vi "_Read CSM Log Filter Rules - v1.0.vi"(7 "Section Name":string="LogFilterRules", 8 "error in (no error)":errorcluster, 11 "LabVIEW-Config.lvlib:LabVIEW-Config.lvclass":refnum<class "LabVIEW-Config.lvclass">) -> (0 "error out":errorcluster, 1 "Rules-v1":T1, 2 "Key Names":string[](array[string]), 3 "Config out":refnum<class "LabVIEW-Config.lvclass">)   [LabVIEW 2017, in "INI-Static-Variable-Support.lvlib"]
uses:
  INI-Static-Variable-Support.lvlib
  LabVIEW-Config/LabVIEW-Config.lvclass
  <userlib>/_NEVSTOP/Communicable State Machine(CSM)/_Support/Typedef/_CSM_GlobalLog Filter Rules - v1.0.ctl
  <userlib>/_NEVSTOP/Communicable State Machine(CSM)/_Support/Typedef/_CSM_GlobalLog_MSG_TYPE.ctl
  <userlib>/_NEVSTOP/Communicable State Machine(CSM)/_Support/Typedef/_CSM_GlobalLog_STATE_TYPE.ctl
  LabVIEW-Config/Read Array Key (String).vi
  <userlib>/_NEVSTOP/Communicable State Machine(CSM)/Communicable State Machine.lvlib
  <userlib>/_NEVSTOP/Communicable State Machine(CSM)/addons/API-String-Arugments-Support/API String Arguments Support.lvlib
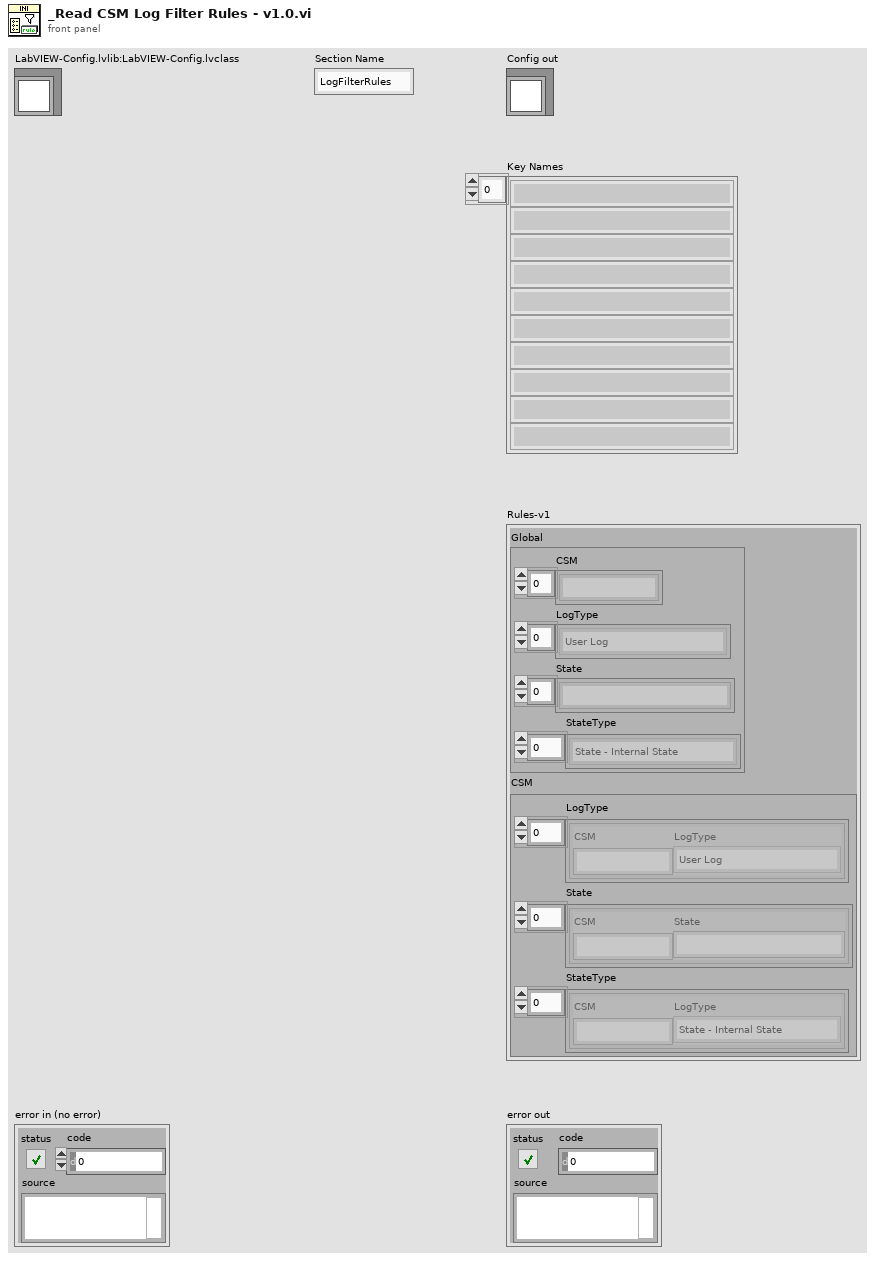
[diagram p1: front panel]
types:
  T1 = typedef "Communicable State Machine.lvlib/_CSM_GlobalLog Filter Rules - v1.0.ctl" = cluster{"Global":cluster{"CSM":string[], "LogType":T2[], "State":string[], "StateType":T3[]}, "CSM":cluster{"LogType":cluster{"CSM":string, "LogType":T2}[], "State":cluster{"CSM":string, "State":string}[], "StateType":cluster{"CSM":string, "LogType":T3}[]}}
  T2 = typedef "Communicable State Machine.lvlib/_CSM_GlobalLog_MSG_TYPE.ctl" = enum16{"User Log", "State Change", "Status", "Interrupt", "Register", "Unregister", "Error Log", "Module Created", "Module Destroyed"}
  T3 = typedef "Communicable State Machine.lvlib/_CSM_GlobalLog_STATE_TYPE.ctl" = enum16{"State - Internal State", "State - External Message", "State - Response", "State - Complete"}
  T4 = cluster{"CSM":string, "CSM_GlobalLog_MSG_TYPE":T2}[]
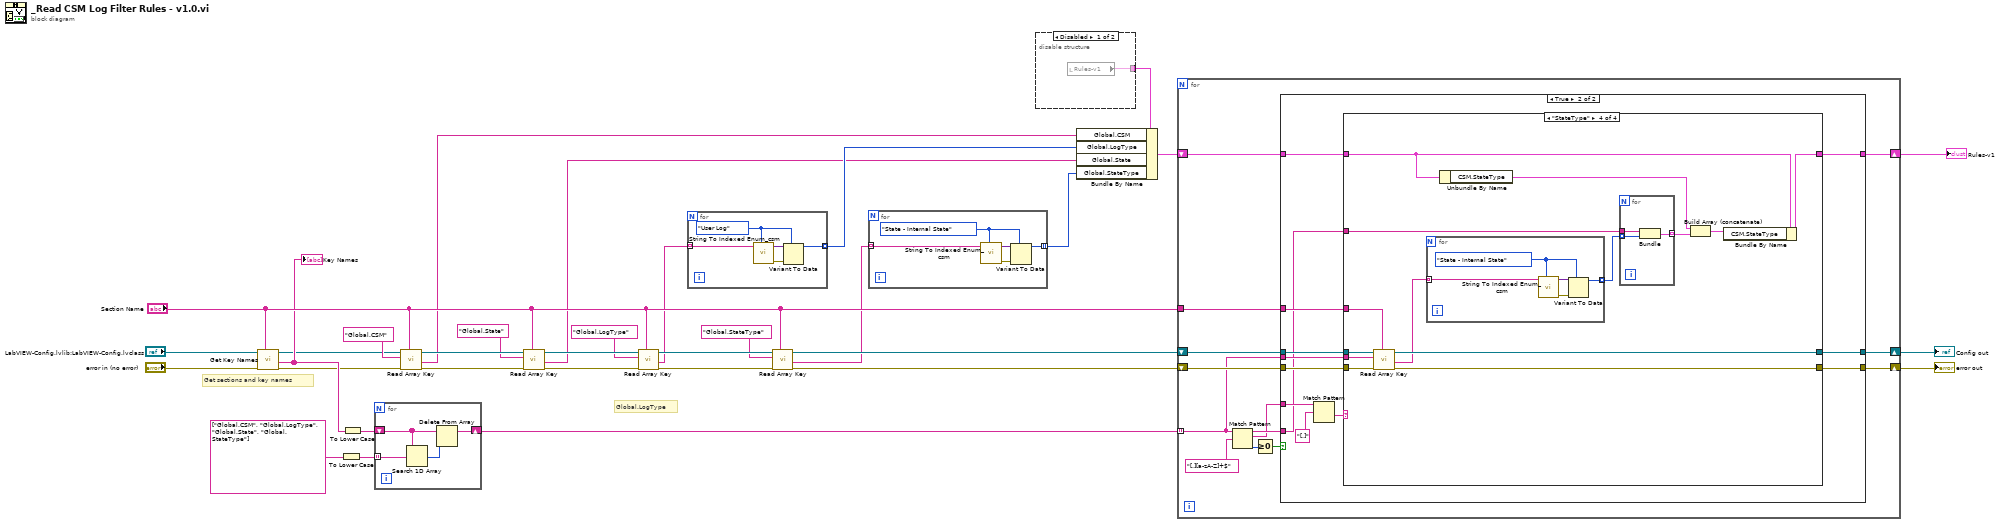
[diagram p0: block diagram]
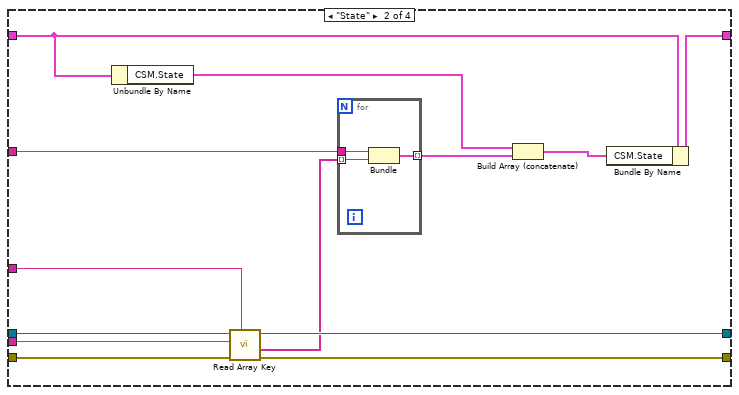
[diagram p5: hidden frame]
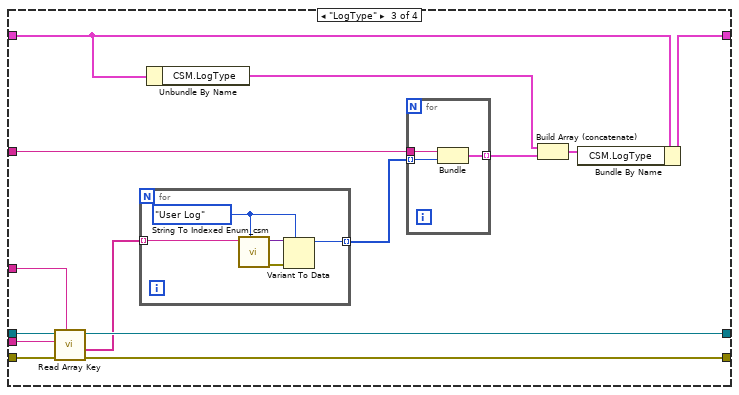
[diagram p6: hidden frame]
diagram:
  # "Global.LogType"
  # "Get sections and key names"
  n1 = call "Get Key Names.vi"("Section Name"="Section Name", "error in (no error)"="error in (no error)", "Config in"="LabVIEW-Config.lvlib:LabVIEW-Config.lvclass") -> ("error out"=w2:errorcluster, "Key Names"=w22:string[], "Config out"=w4:refnum<class "LabVIEW-Config.lvclass">)  [unwired: 5 in, 1 out]
  "Key Names" <- w22
  n2 = To Lower Case(string=string[] ["Global.CSM", "Global.LogType", "Global.State", "Global.StateType"] ("Key Names")) -> (all lower case string=w25:string[])
  n3 = To Lower Case(string=w22) -> (all lower case string=w24:string[])
  n4 = for {
    tunnel: w25 -> [w37] mode=indexing
    shift-right: [w34] -> w28
    shift-left: w24 -> [w36]
    n5 = Search 1D Array(1D array=w36, element=w37) -> (index of element=w35:i32)  [unwired: 1 in]
    n6 = Delete From Array(array=w36, index=w35) -> (array with subset deleted=w34:string[])  [unwired: 1 in, 1 out]
  }
  n7 = call-poly "Read Array Key.vi"("Section Name"="Section Name", "error in (no error)"=w2, "Key Name"="Global.CSM", "Config in"=w4) -> ("error out"=w10:errorcluster, "Value"=w7:string[], "Config out"=w9:refnum<class "LabVIEW-Config.lvclass">)  [unwired: 4 in, 1 out]
  n8 = call-poly "Read Array Key.vi"("Section Name"="Section Name", "error in (no error)"=w10, "Key Name"="Global.State", "Config in"=w9) -> ("error out"=w13:errorcluster, "Value"=w11:string[], "Config out"=w14:refnum<class "LabVIEW-Config.lvclass">)  [unwired: 4 in, 1 out]
  n9 = call-poly "Read Array Key.vi"("Section Name"="Section Name", "error in (no error)"=w13, "Key Name"="Global.LogType", "Config in"=w14) -> ("error out"=w18:errorcluster, "Value"=w16:string[], "Config out"=w19:refnum<class "LabVIEW-Config.lvclass">)  [unwired: 4 in, 1 out]
  n10 = for {
    tunnel: w16 -> [w42] mode=indexing
    tunnel: [w38] -> w17 mode=indexing
    w39 = _CSM_GlobalLog_MSG_TYPE."User Log" ("CSM_GlobalLog_MSG_TYPE")
    n11 = call <userlib>:"String To Indexed Enum_csm.vi"("Variant"=w39, "String"=w42) -> ("error out"=w41:errorcluster, "Enum"=w40:variant)  [unwired: 8 in]
    n12 = Variant To Data(error in=w41, type=w39, Variant=w40) -> (data=w38:T2)  [unwired: 1 out]
  }
  n13 = call-poly "Read Array Key.vi"("Section Name"="Section Name", "error in (no error)"=w18, "Key Name"="Global.StateType", "Config in"=w19) -> ("error out"=w30:errorcluster, "Value"=w20:string[], "Config out"=w29:refnum<class "LabVIEW-Config.lvclass">)  [unwired: 4 in, 1 out]
  n14 = for {
    tunnel: w20 -> [w47] mode=indexing
    tunnel: [w44] -> w21 mode=indexing
    w43 = _CSM_GlobalLog_STATE_TYPE."State - Internal State" ("LogType")
    n15 = call <userlib>:"String To Indexed Enum_csm.vi"("Variant"=w43, "String"=w47) -> ("error out"=w46:errorcluster, "Enum"=w45:variant)  [unwired: 8 in]
    n16 = Variant To Data(error in=w46, type=w43, Variant=w45) -> (data=w44:T3)  [unwired: 1 out]
  }
  n17 = disable-structure "Diagram Disable Structure" shown="Disabled" {
    disable-tunnel: [w48 _] -> w6
    frame Disabled {
      n18 = local read "Rules-v1"() -> (w48:T1)
    }
    frame Enabled {
    }
  }
  n19 = Bundle By Name(cluster=w6, "Global.CSM"=w7, "Global.LogType"=w17, "Global.State"=w11, "Global.StateType"=w21) -> (w26:T1)
  n20 = for {
    shift-right: [w49] -> w27
    shift-left: w26 -> [w56]
    tunnel: w28 -> [w50] mode=indexing
    shift-right: [w51] -> w32
    shift-left: w29 -> [w55]
    shift-right: [w52] -> w33
    shift-left: w30 -> [w54]
    tunnel: "Section Name" -> [w53]
    n21 = Match Pattern(string=w50, regular expression="[.][a-zA-Z]+$") -> (before substring=w58:string, match substring=w57:string, offset past match=w60:i32)  [unwired: 1 in, 1 out]
    n22 = Greater Or Equal To 0?(x=w60) -> (x >= 0?=w59:bool)
    n23 = case shown="True" w59 {
      tunnel: w58 -> [_ w66]
      tunnel: w57 -> [_ w75]
      tunnel: w56 -> [w62 w67]
      tunnel: w55 -> [w64 w73]
      tunnel: w54 -> [w63 w72]
      tunnel: w53 -> [_ w71]
      tunnel: [w63 w70] -> w52
      tunnel: [w64 w69] -> w51
      tunnel: w50 -> [_ w68]
      tunnel: [w62 w65] -> w49
      frame False {
      }
      frame True {
        n24 = Match Pattern(string=w75, regular expression="[.]") -> (after substring=w74:string)  [unwired: 1 in, 3 out]
        n25 = case shown="\"StateType\"" w74 {
          tunnel: w73 -> [w77 w92 w109 w131]
          tunnel: w72 -> [w78 w91 w108 w130]
          tunnel: w71 -> [_ w90 w107 w129]
          tunnel: [w78 w89 w106 w128] -> w70
          tunnel: [w77 w88 w105 w127] -> w69
          tunnel: w68 -> [_ w87 w104 w126]
          tunnel: w67 -> [w79 w82 w98 w120]
          tunnel: w66 -> [_ w85 w103 w125]
          tunnel: [w79 w84 w102 w124] -> w65
          frame Default {
          }
          frame "State" {
            n26 = Unbundle By Name(w82) -> ("CSM.State"=w80:cluster{"CSM":string, "State":string}[])
            n27 = call-poly "Read Array Key.vi"("Section Name"=w90, "error in (no error)"=w91, "Key Name"=w87, "Config in"=w92) -> ("error out"=w89:errorcluster, "Value"=w86:string[], "Config out"=w88:refnum<class "LabVIEW-Config.lvclass">)  [unwired: 4 in, 1 out]
            n28 = for {
              tunnel: w86 -> [w95] mode=indexing
              tunnel: w85 -> [w94]
              tunnel: [w93] -> w83 mode=indexing
              n29 = Bundle(w94, "Value"=w95) -> (w93:cluster{string, "Value":string})  [unwired: 1 in]
            }
            n30 = Build Array (concatenate)(w80, w83) -> (w81:cluster{"CSM":string, "Value":string}[])
            n31 = Bundle By Name(cluster=w82, "CSM.State"=w81) -> (w84:T1)
          }
          frame "LogType" {
            n32 = call-poly "Read Array Key.vi"("Section Name"=w107, "error in (no error)"=w108, "Key Name"=w104, "Config in"=w109) -> ("error out"=w106:errorcluster, "Value"=w100:string[], "Config out"=w105:refnum<class "LabVIEW-Config.lvclass">)  [unwired: 4 in, 1 out]
            n33 = for {
              tunnel: w100 -> [w114] mode=indexing
              tunnel: [w110] -> w99 mode=indexing
              w111 = _CSM_GlobalLog_MSG_TYPE."User Log" ("CSM_GlobalLog_MSG_TYPE")
              n34 = call <userlib>:"String To Indexed Enum_csm.vi"("Variant"=w111, "String"=w114) -> ("error out"=w113:errorcluster, "Enum"=w112:variant)  [unwired: 8 in]
              n35 = Variant To Data(error in=w113, type=w111, Variant=w112) -> (data=w110:T2)  [unwired: 1 out]
            }
            n36 = Unbundle By Name(w98) -> ("CSM.LogType"=w96:cluster{"CSM":string, "LogType":T2}[])
            n37 = for {
              tunnel: w99 -> [w117] mode=indexing
              tunnel: w103 -> [w116]
              tunnel: [w115] -> w101 mode=indexing
              n38 = Bundle(w116, "CSM_GlobalLog_MSG_TYPE"=w117) -> (w115:cluster{string, "CSM_GlobalLog_MSG_TYPE":T2})  [unwired: 1 in]
            }
            n39 = Build Array (concatenate)(w96, w101) -> (w97:T4)
            n40 = Bundle By Name(cluster=w98, "CSM.LogType"=w97) -> (w102:T1)
          }
          frame "StateType" {
            n41 = call-poly "Read Array Key.vi"("Section Name"=w129, "error in (no error)"=w130, "Key Name"=w126, "Config in"=w131) -> ("error out"=w128:errorcluster, "Value"=w121:string[], "Config out"=w127:refnum<class "LabVIEW-Config.lvclass">)  [unwired: 4 in, 1 out]
            n42 = for {
              tunnel: w121 -> [w136] mode=indexing
              tunnel: [w133] -> w122 mode=indexing
              w132 = _CSM_GlobalLog_STATE_TYPE."State - Internal State" ("LogType")
              n43 = call <userlib>:"String To Indexed Enum_csm.vi"("Variant"=w132, "String"=w136) -> ("error out"=w135:errorcluster, "Enum"=w134:variant)  [unwired: 8 in]
              n44 = Variant To Data(error in=w135, type=w132, Variant=w134) -> (data=w133:T3)  [unwired: 1 out]
            }
            n45 = Unbundle By Name(w120) -> ("CSM.StateType"=w118:cluster{"CSM":string, "LogType":T3}[])
            n46 = for {
              tunnel: w122 -> [w139] mode=indexing
              tunnel: w125 -> [w138]
              tunnel: [w137] -> w123 mode=indexing
              n47 = Bundle(w138, "LogType"=w139) -> (w137:cluster{string, "LogType":T3})  [unwired: 1 in]
            }
            n48 = Build Array (concatenate)(w118, w123) -> (w119:cluster{"CSM":string, "LogType":T3}[])
            n49 = Bundle By Name(cluster=w120, "CSM.StateType"=w119) -> (w124:T1)
          }
        }
      }
    }
  }
  "error out" <- w33
  "Config out" <- w32
  "Rules-v1" <- w27
